vi "add_to_arr.vi"(10 "item":dbl, 11 "array":dbl[](array[numeric])) -> (3 "result_array":dbl[](array[numeric]))   [LabVIEW 2017]
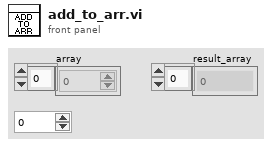
[diagram p1: front panel]
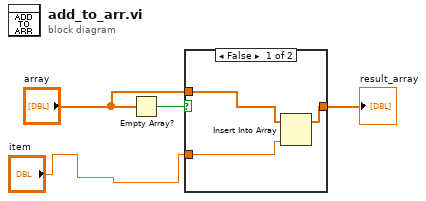
[diagram p0: block diagram]
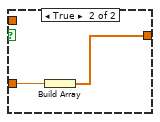
[diagram p2: hidden frame]
diagram:
  n1 = Empty Array?(array="array") -> (empty?=w3:bool)
  n2 = case shown="False" w3 {
    tunnel: "item" -> [w7 w9]
    tunnel: "array" -> [w6 _]
    tunnel: [w5 w8] -> w1
    frame False {
      n3 = Insert Into Array(array=w6, new element=w7) -> (w5:dbl[])  [unwired: 1 in]
    }
    frame True {
      n4 = Build Array(w9) -> (w8:dbl[])
    }
  }
  "result_array" <- w1
